vi "Soll Ist Vergleich wet.vi"(6 "Enum":T1, 8 "error in (no error)":errorcluster caption="Fehler (Eingang, kein Fehler)", 9 "Toleranz":sgl, 10 "Ist":sgl, 11 "Soll":sgl) -> (0 "error out":errorcluster caption="Fehler (Ausgang)", 1 "Erreicht":bool, 2 "Erreicht 10Sek":bool, 3 "Fehler %":dbl)   [LabVIEW 2015]
uses:
  Aktion Soll Ist.ctl
  Interference verificaton 1065-366.lvlib
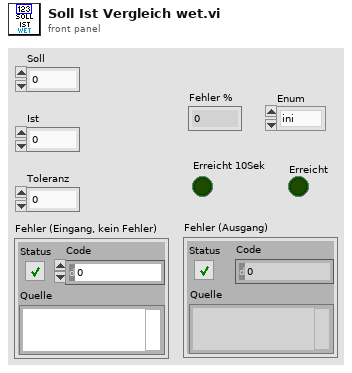
[diagram p1: front panel]
types:
  T1 = typedef "EPA 1065.lvlib/Interference verificaton 1065-366.lvlib/Aktion Soll Ist.ctl" = enum16{"ini", "run"}
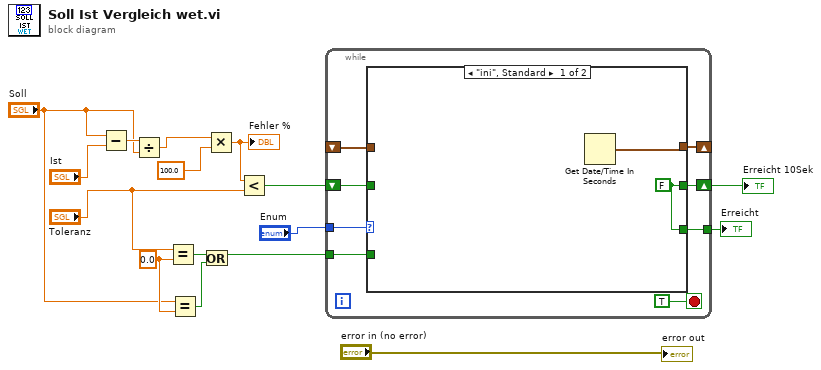
[diagram p0: block diagram]
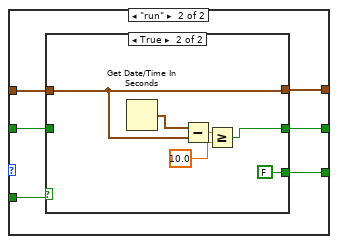
[diagram p2: hidden frame]
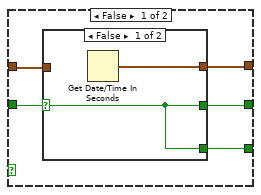
[diagram p3: hidden frame]
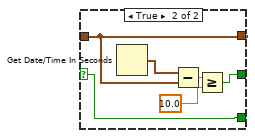
[diagram p4: hidden frame]
diagram:
  w6 = sgl 0.0 ("y")
  n1 = Subtract(x="Soll", y="Ist") -> (x-y=w15:sgl)
  n2 = Divide(x=w15, y="Soll") -> (x/y=w2:sgl)
  n3 = Equal?(x="Toleranz", y=w6) -> (x = y?=w7:bool)
  n4 = Equal?(x="Soll", y=w6) -> (x = y?=w4:bool)
  n5 = Or(x=w7, y=w4) -> (x .or. y?=w5:bool)
  n6 = Multiply(x=w2, y=100.0 ("x")) -> (x*y=w10:dbl)
  "Fehler %" <- w10
  n7 = Less?(x=w10, y="Toleranz") -> (x < y?=w14:bool)
  n8 = while {
    shift-right: [w22] -> w13
    shift-left: w14 -> [w23]
    shift-right: [w21] -> _
    shift-left: _ -> [w20]
    tunnel: "Enum" -> [w19]
    tunnel: w5 -> [w18]
    tunnel: [w17] -> w1
    stop <- TRUE stop-if-true
    n9 = case shown="\"ini\", Standard" w19 {
      tunnel: w23 -> [_ w32]
      tunnel: [w25 w31] -> w22
      tunnel: [w26 w30] -> w21
      tunnel: w20 -> [_ w29]
      tunnel: w18 -> [_ w28]
      tunnel: [w25 w27] -> w17
      frame "ini", Default {
        w25 = FALSE
        n10 = Get Date/Time In Seconds() -> (seconds since 1Jan1904=w26:timestamp)
      }
      frame "run" {
        n11 = case shown="True" w28 {
          tunnel: w32 -> [w37 _]
          tunnel: [w36 w48] -> w31
          tunnel: [w35 w47] -> w30
          tunnel: w29 -> [w34 w47]
          tunnel: [w33 FALSE] -> w27
          frame False {
            n12 = case shown="False" w37 {
              selector: w37 -> [w38 w40]
              tunnel: [w38 w42] -> w36
              tunnel: [w39 w41] -> w35
              tunnel: w34 -> [_ w41]
              tunnel: [w38 w40] -> w33
              frame False {
                n13 = Get Date/Time In Seconds() -> (seconds since 1Jan1904=w39:timestamp)
              }
              frame True {
                n14 = Get Date/Time In Seconds() -> (seconds since 1Jan1904=w43:timestamp)
                n15 = Subtract(x=w43, y=w41) -> (x-y=w45:dbl)
                n16 = Greater Or Equal?(x=w45, y=10.0) -> (x >= y?=w42:bool)
              }
            }
          }
          frame True {
            n17 = Get Date/Time In Seconds() -> (seconds since 1Jan1904=w49:timestamp)
            n18 = Subtract(x=w49, y=w47) -> (x-y=w51:dbl)
            n19 = Greater Or Equal?(x=w51, y=10.0) -> (x >= y?=w48:bool)
          }
        }
      }
    }
  }
  "Erreicht 10Sek" <- w13
  "Erreicht" <- w1
  "error out" <- "error in (no error)"
